vi "Test Referencing.vi"() -> ()   [LabVIEW 2013]
panel:
  in  "Z Stage Serial":i32
  in  "Z Stage Motor":refnum<k7>(container)
  in  "Y Stage Serial":i32
  in  "Y Stage Motor":refnum<k7>(container)
  in  "X Stage Serial":i32
  in  "X Stage motor":refnum<k7>(container)
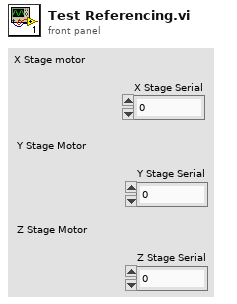
[diagram p1: front panel]
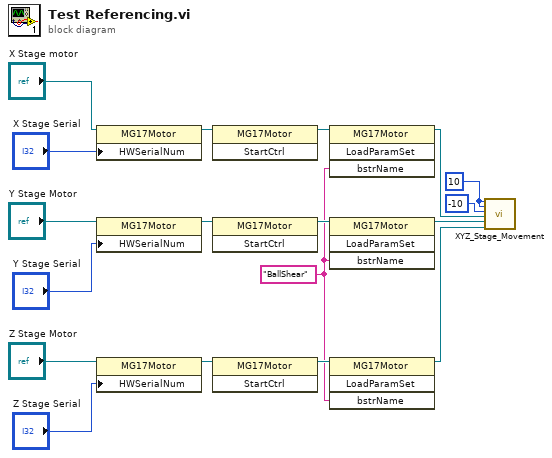
[diagram p0: block diagram]
diagram:
  w1 = 10
  w3 = "BallShear"
  n1 = property class="MG17Motor"(reference="X Stage motor", "HWSerialNum"="X Stage Serial") -> (reference out=w17:refnum<k7>)  [unwired: 1 in, 1 out]
  n2 = property class="MG17Motor"(reference="Y Stage Motor", "HWSerialNum"="Y Stage Serial") -> (reference out=w14:refnum<k7>)  [unwired: 1 in, 1 out]
  n3 = property class="MG17Motor"(reference="Z Stage Motor", "HWSerialNum"="Z Stage Serial") -> (reference out=w11:refnum<k7>)  [unwired: 1 in, 1 out]
  n4 = invoke class="MG17Motor" method="StartCtrl"(reference=w17) -> (reference out=w16:refnum<k7>)  [unwired: 2 in, 2 out]
  n5 = invoke class="MG17Motor" method="StartCtrl"(reference=w14) -> (reference out=w13:refnum<k7>)  [unwired: 2 in, 2 out]
  n6 = invoke class="MG17Motor" method="StartCtrl"(reference=w11) -> (reference out=w10:refnum<k7>)  [unwired: 2 in, 2 out]
  n7 = invoke class="MG17Motor" method="LoadParamSet"(reference=w16, "bstrName"=w3) -> (reference out=w9:refnum<k7>)  [unwired: 2 in, 3 out]
  n8 = invoke class="MG17Motor" method="LoadParamSet"(reference=w13, "bstrName"=w3) -> (reference out=w8:refnum<k7>)  [unwired: 2 in, 3 out]
  n9 = invoke class="MG17Motor" method="LoadParamSet"(reference=w10, "bstrName"=w3) -> (reference out=w7:refnum<k7>)  [unwired: 2 in, 3 out]
  n10 = call "XYZ_Stage_Movement.vi"("X Input"=w1, "Y Input"=w1, "Z Input"=-10, "X Ref"=w9, "Y Ref"=w8, "Z Ref"=w7) -> ()  [unwired: 11 in, 3 out]
